vi "Gage_Set.vi"(7 "Scope":bool, 10 "Handle Cluster 2":T1, 11 "Handle Cluster 1":T1) -> (0 "Waveform Graph":cluster{i32, dbl, dbl[]}(graph), 1 "Equivalent RT delay\ndistance (mm)":dbl=1.5 format="%.4f")   [LabVIEW 2022 SP3]
uses:
  <vilib>/Analysis/NI_AALPro.lvlib
  -GageUtils/GageGlobals.vi
  <vilib>/Utility/file.llb/Write To Spreadsheet File (DBL).vi
  <vilib>/Analysis/NI_AALBase.lvlib
  <vilib>/Analysis/baseanly.llb/Mean (DBL).vi
panel:
  in  "Slave scales":bool
  in  "holdoff (ms)":dbl min=0.0
  out "Gage Chan 9-16":dbl[][](graph)
  out "LeCroy Ch1":dbl[](graph)
  in  "Set LeCroy":bool
  in  "time out (ms)":dbl=1000.0 min=-1.0
  in  "Vpp Chs 2":i16[](array[ring])=[5, 5, 5, 5, 5, 5, 5, 5]
  in  "Ch":u16 max=15
  out "Status":string
  in  "Mode":u16(ring)=3 items=["Single", "Dual", "Quad", "Octal"]
  in  "Coupling":u16(ring) items=["DC", "AC"]
  in  "Impedance":u32=50 min=50 max=1000000 step=999950
  out "Nominal Samples":i32
  out "t per div":dbl
  in  "Vpp Chs 1":i16[](array[ring])=[5, 5, 5, 5, 5, 5, 5, 5]
  out "Gage Chan 1-8":dbl[][](graph)
  in  "Save trace?":bool
  out "Total Delay (ms)":dbl=1.5 format="%.3f"
  in  "go to scan type":bool
  in  "ExitSendCmd":bool
  in  "Time scale per Div":i32(ring)=1 items=["1 micros", "2 micros", "5 micros", "10 micros", "20 micros", "50 micros", "100 micros", "200 micros", "500 micros", "1 ms", "2 ms", "5 ms", "10 ms"]
  in  "Trigger Settings":T2={"Trig Source"=1, "Level (%)"=25.0, "External"=TRUE, "Ext Impedance"=1, "External Coupling"=0, "Ext Trig Range"=0, "Slope"=0} {"Slope" items=["Rising", "Falling"]; "Ext Trig Range" items=["+/- 5 Volts", "+/- 1 Volt"]; "External Coupling" items=["DC", "AC"]; "Ext Impedance" items=["50 Ohm", "HiZ"]; "Level (%)" min=-100.0 max=100.0 format="%#.2f"; "Trig Source" items=["Ch 0", "Ch 1", "Ch 2", "Ch 3", "Ch 4", "Ch 5", "Ch 6", "Ch 7"]}
  in  "RF data Sampling":T3={"Sampling Rate"=6, "Ref Delay (ms)"=0.0, "rf points per line"=2048} {"Sampling Rate" items=["1 MS/s", "5 MS/s", "10 MS/s", "25 MS/s", "50 MS/s", "100 MS/s", "125 MS/s"]; "Ref Delay (ms)" min=0.0 format="%.2f"}
  # "Digitizer Settings"
  # "Scale Settings"
  # "Yellow curser used for additional delay. RF data is captured between yellow and red lines."
  # "Scope sampling rate should be fixed at 250 MS/s"
  # "© 2009 Riverside Research Institute"
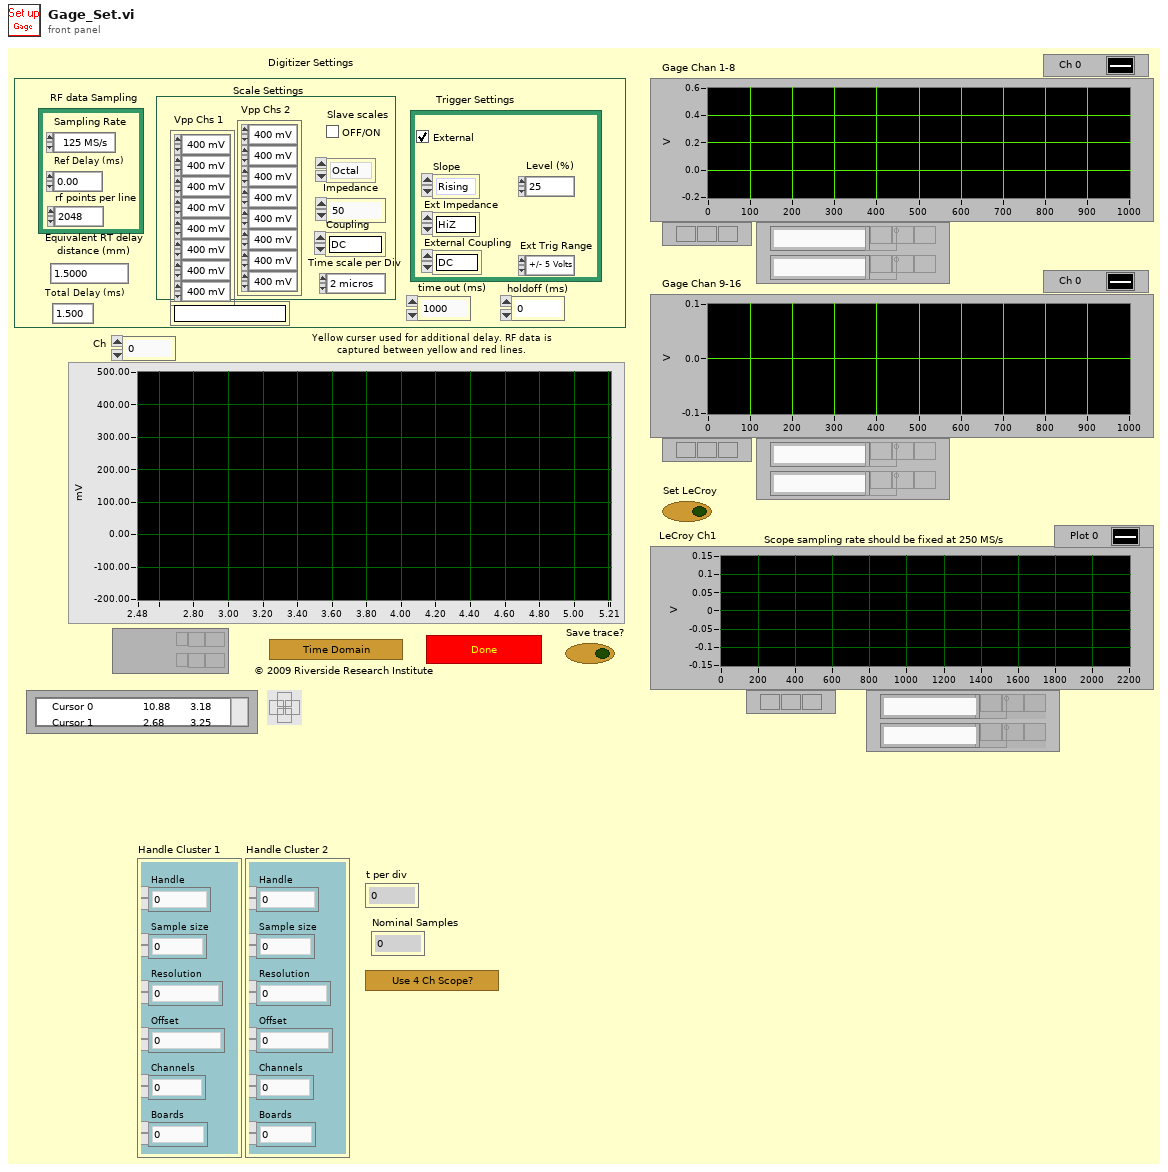
[diagram p1: front panel]
types:
  T1 = cluster{"Handle":u32, "Sample size":u32, "Resolution":i32, "Offset":i32, "Channels":u32, "Boards":u32}
  T2 = cluster{"Trig Source":u16, "Level (%)":dbl, "External":bool, "Ext Impedance":u16, "External Coupling":u16, "Ext Trig Range":i16, "Slope":u16}
  T3 = cluster{"Sampling Rate":u16, "Ref Delay (ms)":dbl, "rf points per line":i32}
  T4 = cluster{"Handle":u32, "Sample Size":u32, "Resolution":i32, "Offset":i32, "Channels":u32, "Boards":u32}
  T5 = cluster{dbl, "Clock mode":enum16{"Internal", "External", "Reference"}, "RingText.Text":string, i32, i32, "time out (ms)":dbl, dbl, dbl}
  T6 = cluster{"RingText.Text":string, bool, bool, i16, "Impedance":u32, i32, i32}
  T7 = cluster{"RingText.Text":string, "Level (%)":dbl, "Trig Source":u16, i32, "RingText.Text":string, "External":bool, bool, "RingText.Text":string}
  T8 = cluster{"RingText.Text":string, "Level (%)":dbl, "Trig Source":u16, i32, "RingText.Text":string, "External":bool, bool, "RingText.Text":string}[]
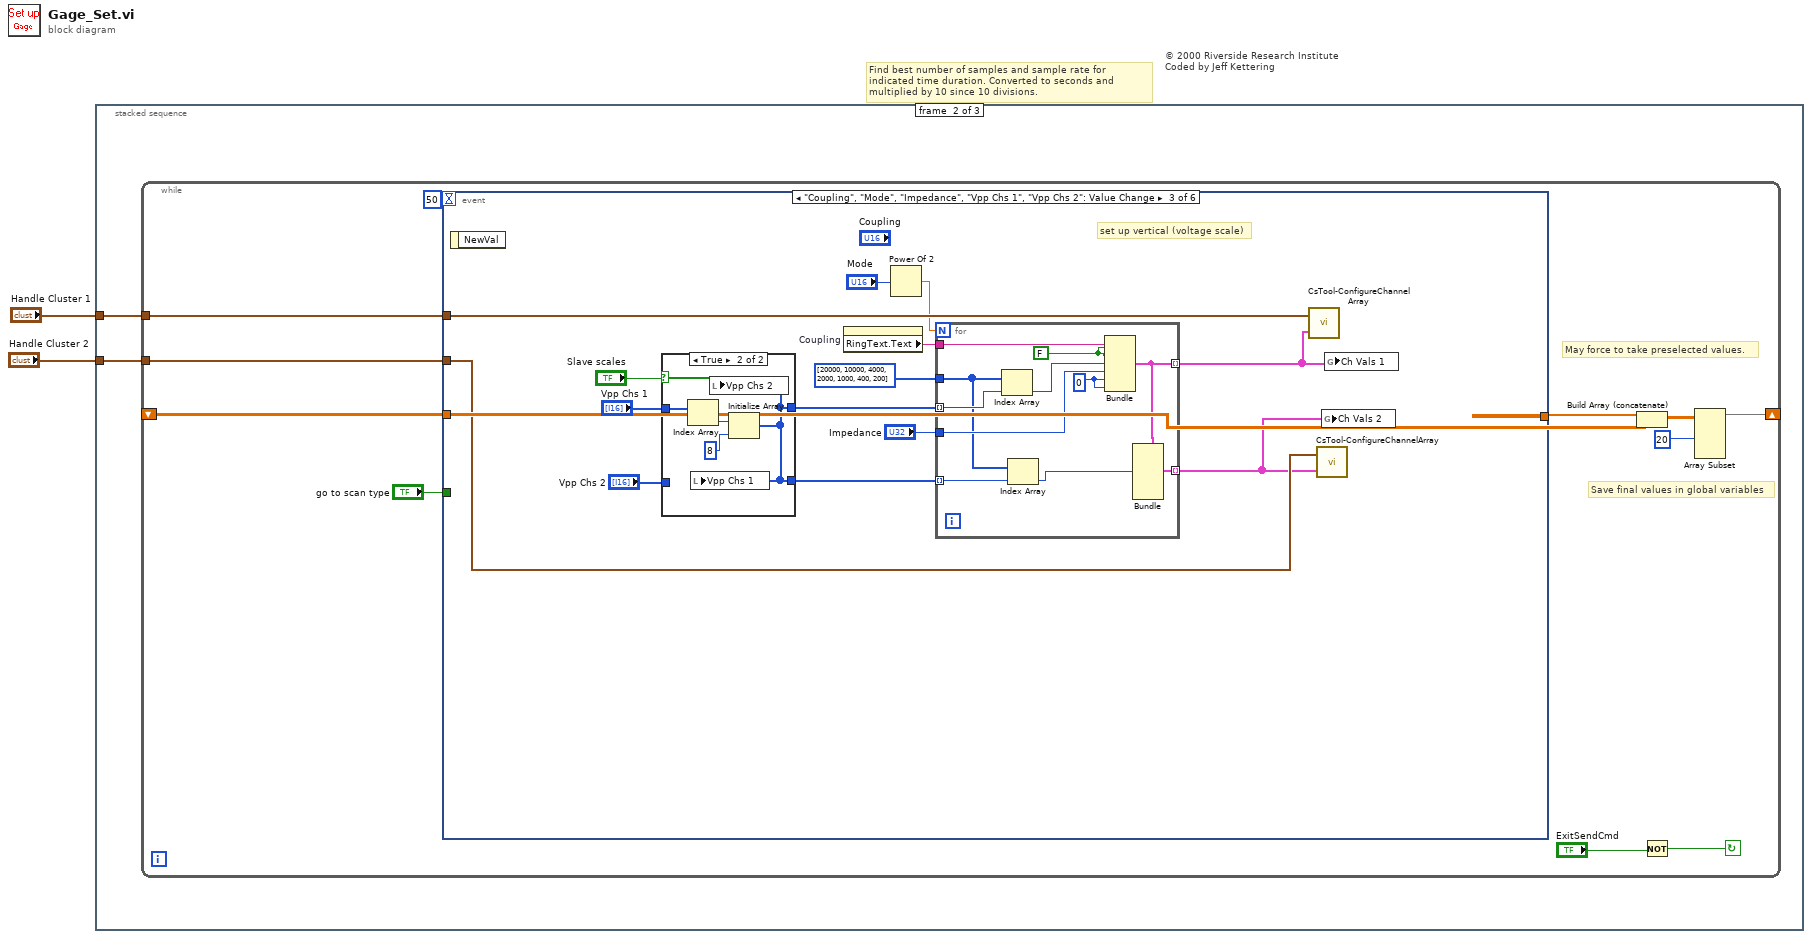
[diagram p0: block diagram]
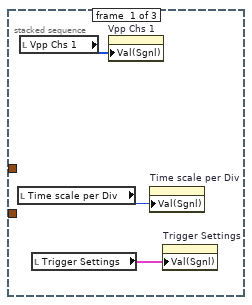
[diagram p2: hidden frame]
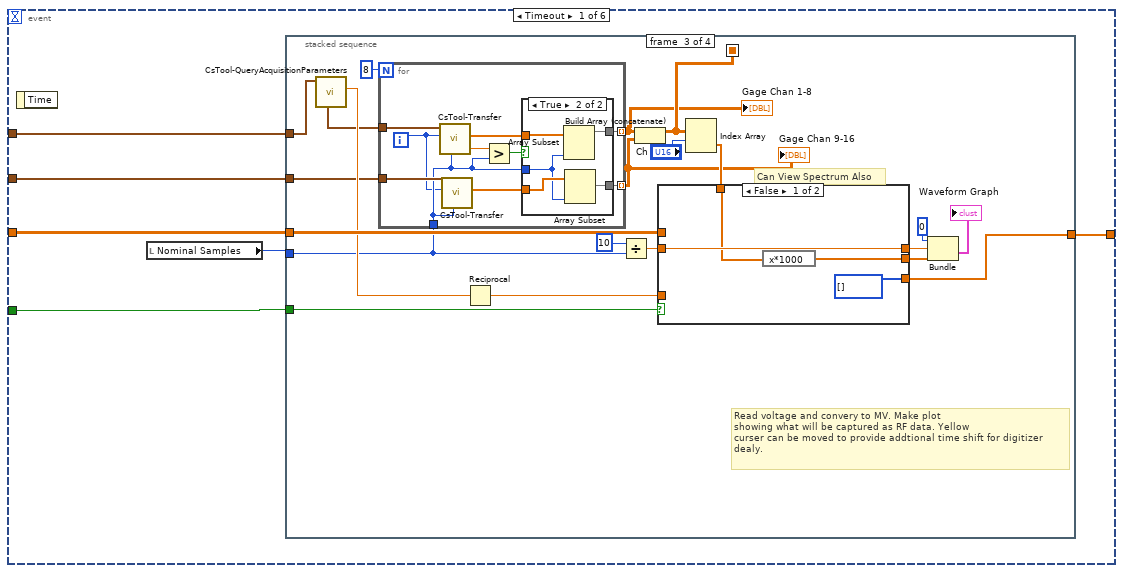
[diagram p3: hidden frame]
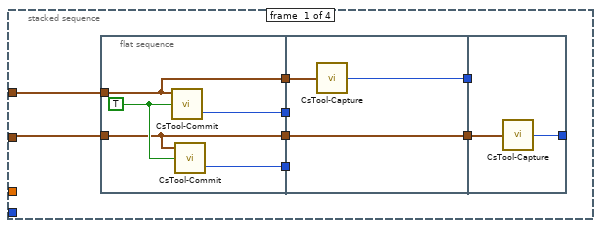
[diagram p4: hidden frame]
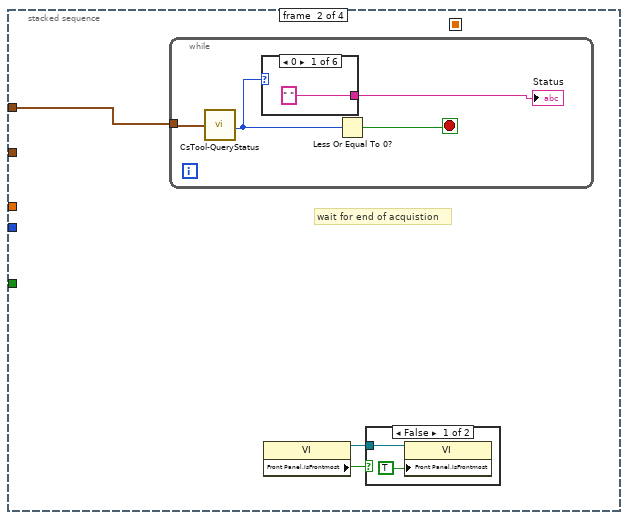
[diagram p5: hidden frame]
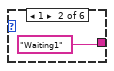
[diagram p6: hidden frame]
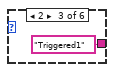
[diagram p7: hidden frame]
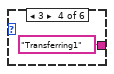
[diagram p8: hidden frame]
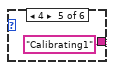
[diagram p9: hidden frame]
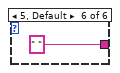
[diagram p10: hidden frame]
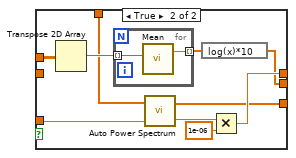
[diagram p13: hidden frame]
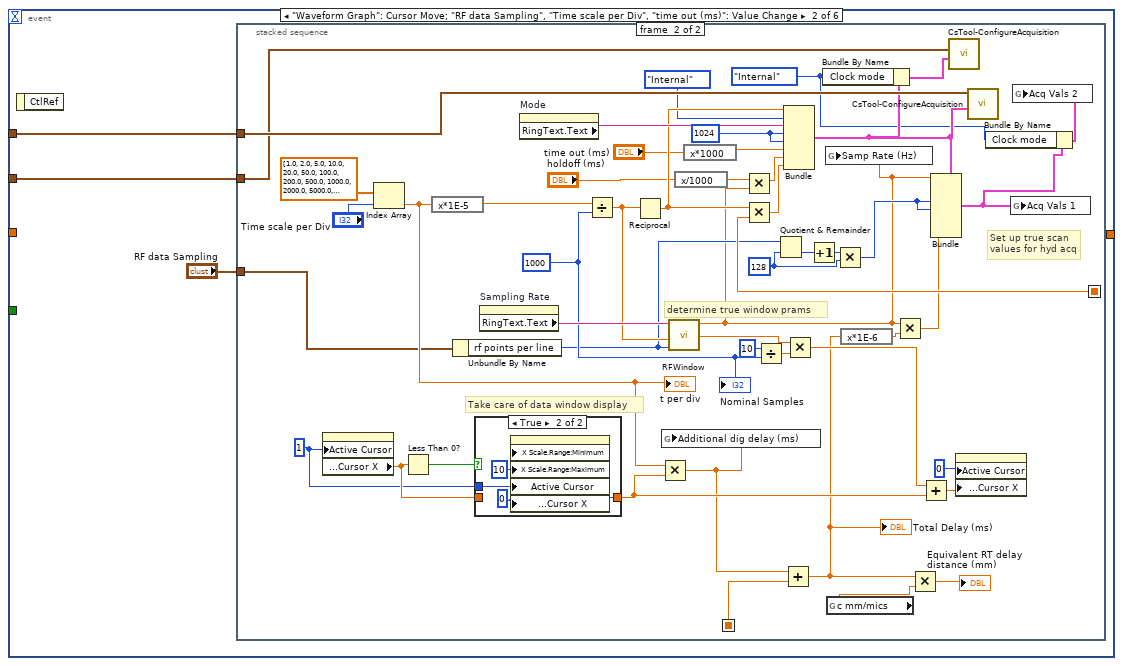
[diagram p15: hidden frame]
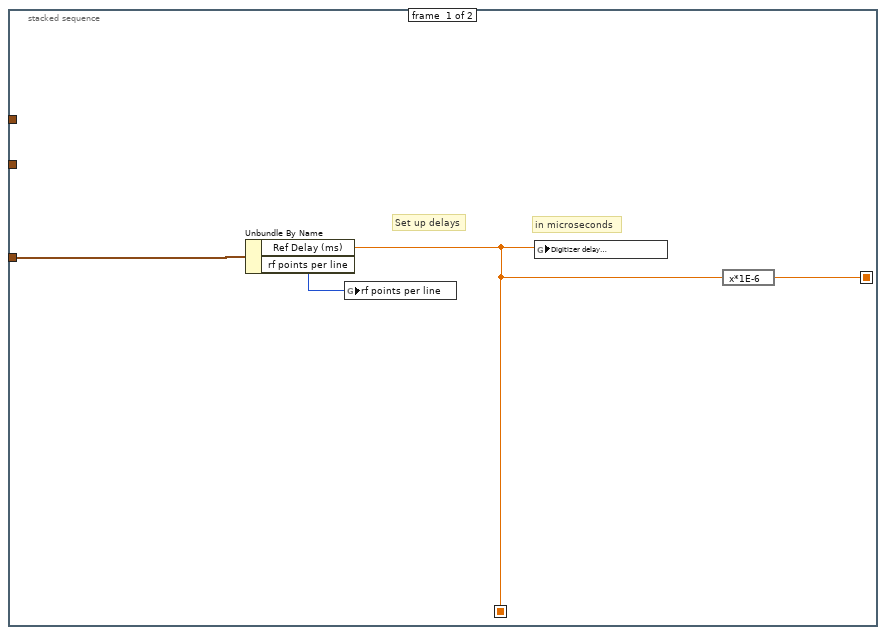
[diagram p16: hidden frame]
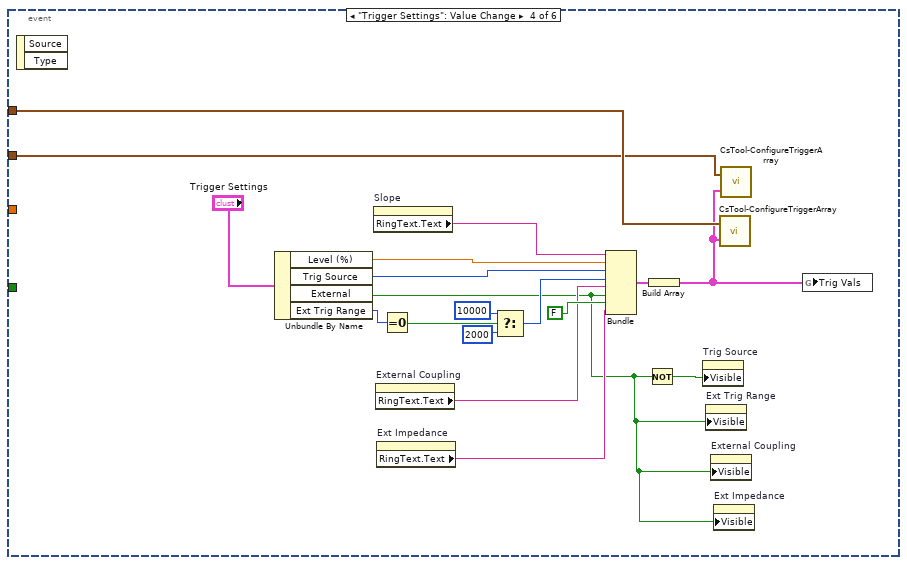
[diagram p19: hidden frame]
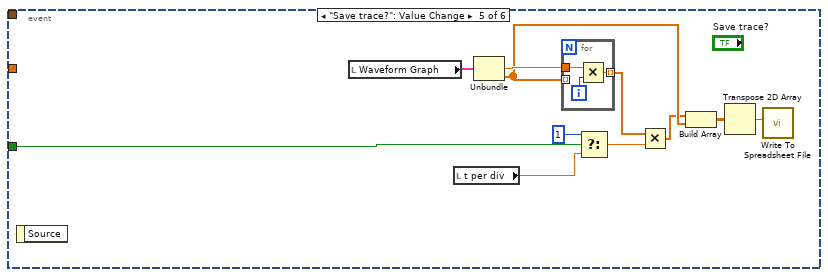
[diagram p20: hidden frame]
diagram:
  # "Find best number of samples and sample rate for indicated time duration. Converted to seconds and multiplied by 10 since 10 divisions."
  # "© 2000 Riverside Research Institute\nCoded by Jeff Kettering"
  n1 = stacked-sequence {
    tunnel: "Handle Cluster 1" -> [_ w7 _]
    tunnel: "Handle Cluster 2" -> [_ w6 _]
    frame #0 {
      n2 = local read "Time scale per Div"() -> (w4:i32)
      n3 = local read "Vpp Chs 1"() -> (w5:i16[])
      n4 = local read "Trigger Settings"() -> (w3:T2)
      n5 = property on="Vpp Chs 1" class="Arr (strict)"("Val(Sgnl)"=w5) -> ()  [unwired: 2 in, 2 out]
      n6 = property on="Time scale per Div" class="Ring (strict)"("Val(Sgnl)"=w4) -> ()  [unwired: 2 in, 2 out]
      n7 = property on="Trigger Settings" class="Clust (strict)"("Val(Sgnl)"=w3) -> ()  [unwired: 2 in, 2 out]
    }
    frame #1 {
      n8 = while {
        shift-left: _ -> [w9]
        shift-right: [w14] -> _
        tunnel: w7 -> [w11]
        tunnel: w6 -> [w8]
        stop <- w17 continue-if-true
        # "May force to take preselected values."
        # "Save final values in global variables"
        n9 = event shown="[2] \"Coupling\", \"Mode\", \"Impedance\", \"Vpp Chs 1\", \"Vpp Chs 2\": Value Change" {
          selector: _ -> [_ _ _ _ _ _]
          dyn-events: _ -> [_ _ _ _ _ _]
          timeout: 50 -> [_ _ _ _ _ _]
          tunnel: "go to scan type" -> [w22 _ _ _ w223 _]
          tunnel: w11 -> [w21 w114 w185 w219 _ _]
          tunnel: w9 -> [w24 _ _ _ _ _]
          tunnel: [w23 _ _ _ _ _] -> w16
          tunnel: w8 -> [w19 w112 w178 w205 _ _]
          event Timeout {
            n10 = event-data() -> ()  [unwired: 2 out]
            n11 = local read "Nominal Samples"() -> (w20:i32)
            n12 = stacked-sequence {
              seq-local: [_ _ w61 _] -> [_ _ _ _]
              tunnel: w21 -> [w32 w43 w64 _]
              tunnel: w24 -> [_ _ w73 _]
              tunnel: [_ _ w72 _] -> w23
              tunnel: w22 -> [_ _ w71 _]
              tunnel: w20 -> [_ _ w65 _]
              tunnel: w19 -> [w26 _ w60 _]
              frame #0 {
                n13 = flat-sequence {
                  tunnel: w32 -> [w35]
                  tunnel: [w35] -> w31
                  tunnel: [w37] -> w30
                  tunnel: [w36] -> w29
                  tunnel: [w33] -> w27
                  tunnel: w26 -> [w33]
                  tunnel: w31 -> [w40]
                  tunnel: w30 -> [_]
                  tunnel: w29 -> [_]
                  tunnel: [w39] -> w28
                  tunnel: w27 -> [w39]
                  tunnel: [w38] -> w25
                  tunnel: w28 -> [w42]
                  tunnel: w25 -> [_]
                  tunnel: [w41] -> _
                  frame #0 {
                    w34 = TRUE ("Coerce Flag (f)")
                    n14 = call <userlib>:"CsTool-Commit.vi"("Coerce Flag (f)"=w34, "Handle Cluster"=w35) -> ("Error Code"=w37:i32)  [unwired: 1 in, 1 out]
                    n15 = call <userlib>:"CsTool-Commit.vi"("Coerce Flag (f)"=w34, "Handle Cluster"=w33) -> ("Error Code"=w36:i32)  [unwired: 1 in, 1 out]
                  }
                  frame #1 {
                    n16 = call <userlib>:"CsTool-Capture.vi"("Handle Cluster"=w40) -> ("Error Code"=w38:i32)
                  }
                  frame #2 {
                    n17 = call <userlib>:"CsTool-Capture.vi"("Handle Cluster"=w42) -> ("Error Code"=w41:i32)
                  }
                }
              }
              frame #1 {
                # "wait for end of acquistion"
                n18 = while {
                  tunnel: w43 -> [w48]
                  stop <- w47 stop-if-true
                  n19 = call <userlib>:"CsTool-QueryStatus.vi"("Handle Cluster"=w48) -> ("Status"=w49:i32)
                  n20 = case shown="0" w49 {
                    tunnel: [" " "Waiting1" "Triggered1" "Transferring1" "Calibrating1" " "] -> w46
                    frame 0 {
                    }
                    frame 1 {
                    }
                    frame 2 {
                    }
                    frame 3 {
                    }
                    frame 4 {
                    }
                    frame 5, Default {
                    }
                  }
                  "Status" <- w46
                  n21 = Less Or Equal To 0?(x=w49) -> (x <= 0?=w47:bool)
                }
                n22 = property class="VI"() -> (reference out=w45:refnum<vi>, "Front Panel.IsFrontmost"=w44:bool)  [unwired: 2 in, 1 out]
                n23 = case shown="False" w44 {
                  tunnel: w45 -> [w57 _]
                  frame False {
                    n24 = property class="VI"(reference=w57, "Front Panel.IsFrontmost"=TRUE) -> ()  [unwired: 1 in, 2 out]
                  }
                  frame True {
                  }
                }
              }
              frame #2 {
                # "Can View Spectrum Also"
                # "Read voltage and convery to MV. Make plot\nshowing what will be captured as RF data. Yellow\ncurser can be moved to provide addtional time shift for digitizer\ndealy."
                n25 = call <userlib>:"CsTool-QueryAcquisitionParameters.vi"("Handle Cluster"=w64) -> ("Output Handle Cluster"=w63:T4, "Sample Rate"=w67:dbl)  [unwired: 9 out]
                n26 = for {
                  N: 8 -> [_]
                  tunnel: [w87] -> w59 mode=indexing
                  tunnel: w63 -> [w86]
                  tunnel: w65 -> [w83]
                  tunnel: w60 -> [w84]
                  tunnel: [w82] -> w58 mode=indexing
                  i -> [w81]
                  n27 = call <userlib>:"CsTool-Transfer.vi"("Length (4096)"=w83, "Channel (0)"=w81, "Handle Cluster"=w86) -> ("Actual Length"=w85:dbl, "Data in Volts"=w79:dbl[])  [unwired: 3 in, 2 out]
                  n28 = call <userlib>:"CsTool-Transfer.vi"("Length (4096)"=w83, "Channel (0)"=w81, "Handle Cluster"=w84) -> ("Data in Volts"=w80:dbl[])  [unwired: 3 in, 3 out]
                  n29 = Greater?(x=w85, y=w83) -> (0:w88:bool)
                  n30 = case shown="True" w88 {
                    tunnel: w79 -> [w90 w95]
                    tunnel: [w90 w94] -> w87
                    tunnel: w83 -> [_ w91]
                    tunnel: w80 -> [w89 w93]
                    tunnel: [w89 w92] -> w82
                    frame False {
                    }
                    frame True {
                      n31 = Array Subset(array=w95, length=w91) -> (w94:dbl[])  [unwired: 1 in]
                      n32 = Array Subset(array=w93, length=w91) -> (w92:dbl[])  [unwired: 1 in]
                    }
                  }
                }
                "Gage Chan 1-8" <- w59
                "Gage Chan 9-16" <- w58
                n33 = Reciprocal(x=w67) -> (1/x=w66:dbl)
                n34 = Divide(x=10, y=w65) -> (x/y=w75:dbl)
                n35 = Build Array (concatenate)(w59, w58) -> (w61:dbl[][])
                n36 = Index Array(array=w61, index (row)="Ch") -> (element=w68:dbl[])  [unwired: 1 in]
                n37 = case shown="False" w71 {
                  tunnel: [w96 w101] -> w70
                  tunnel: w68 -> [w97 w107]
                  tunnel: [w99 w103] -> w76
                  tunnel: w75 -> [w99 _]
                  tunnel: w73 -> [_ w106]
                  tunnel: w66 -> [_ w105]
                  tunnel: [i32[] [] w102] -> w72
                  frame False {
                    n38 = expression code="x*1000"(w97) -> (w96:dbl[])
                  }
                  frame True {
                    n39 = Transpose 2D Array(2D array=w106) -> (transposed array=w108:dbl[][])
                    n40 = for {
                      tunnel: w108 -> [w111] mode=indexing
                      tunnel: [w110] -> w100 mode=indexing
                      n41 = call-poly <vilib>:"Mean.vi"("X"=w111) -> ("mean"=w110:dbl)  [unwired: 1 out]
                    }
                    n42 = call <vilib>:"Auto Power Spectrum.vi"("dt"=w105, "Signal (V)"=w107) -> ("df"=w104:dbl, "Power Spectrum (V^2 rms)"=w102:dbl[])
                    n43 = expression code="log(x)*10"(w100) -> (w101:dbl[])
                    n44 = Multiply(x=w104, y=1e-06) -> (x*y=w103:dbl)
                  }
                }
                n45 = Bundle(0, w76, w70) -> (→"Waveform Graph":cluster{i32, dbl, dbl[]})  [unwired: 1 out]
              }
              frame #3 {
                # "May need to alter display to break into subplots"
              }
            }
          }
          event "Waveform Graph": Cursor Move; "RF data Sampling", "Time scale per Div", "time out (ms)": Value Change {
            n46 = event-data() -> ()  [unwired: 2 out]
            n47 = stacked-sequence {
              seq-local: [w118 _] -> [_ w145]
              seq-local: [w116 _] -> [_ w157]
              tunnel: w114 -> [_ w148]
              tunnel: "RF data Sampling" -> [w117 w152]
              tunnel: w112 -> [_ w133]
              frame #0 {
                # "Set up delays"
                # "in microseconds"
                n48 = Unbundle By Name(w117) -> ("Ref Delay (ms)"=w116:dbl, "rf points per line"=w115:i32)
                n49 = global write "GageGlobals.vi" "rf points per line"(w115) -> ()
                n50 = global write "GageGlobals.vi" "Digitizer delay\n (ms)"(w116) -> ()
                n51 = expression code="x*1E-6"(w116) -> (w118:dbl)
              }
              frame #1 {
                w124 = enum16{"Internal", "External", "Reference"}."Internal" ("Clock mode")
                w137 = 128
                w144 = 1024
                w143 = 1000
                w163 = u32 1 ("Write Attribute")
                # "determine true window prams"
                # "Set up true scan values for hyd acq"
                # "Take care of data window display"
                n52 = property on="Waveform Graph" class="WFGraph (strict)"("Active Cursor"=w163) -> ("Cursor.Cursor Position:Cursor X"=w165:dbl)  [unwired: 2 in, 2 out]
                n53 = Index Array(array=dbl[] [1.0, 2.0, 5.0, 10.0, 20.0, 50.0, 100.0, 200.0, 500.0, 1000.0, 2000.0, 5000.0, 10000.0, 20000.0, 50000.0, 100000.0], index="Time scale per Div") -> (element=w154:dbl)
                "t per div" <- w154
                n54 = Less Than 0?(x=w165) -> (x < 0?=w164:bool)
                n55 = expression code="x*1E-5"(w154) -> (w150:dbl)
                n56 = Unbundle By Name(w152) -> ("rf points per line"=w135:i32)
                n57 = case shown="True" w164 {
                  tunnel: w165 -> [w168 _]
                  tunnel: [w168 w169] -> w160
                  tunnel: w163 -> [_ w171]
                  frame False {
                  }
                  frame True {
                    w169 = 0
                    n58 = property on="Waveform Graph" class="WFGraph (strict)"("X Scale.Range:Minimum"=w169, "X Scale.Range:Maximum"=10, "Active Cursor"=w171, "Cursor.Cursor Position:Cursor X"=w169) -> ()  [unwired: 2 in, 2 out]
                  }
                }
                n59 = property on="Sampling Rate" class="Ring (strict)"() -> ("RingText.Text"=w151:string)  [unwired: 2 in, 2 out]
                n60 = property on="Mode" class="Ring (strict)"() -> ("RingText.Text"=w147:string)  [unwired: 2 in, 2 out]
                n61 = Divide(x=w150, y=w143) -> (x/y=w149:dbl)
                n62 = Reciprocal(x=w149) -> (1/x=w142:dbl)
                n63 = Multiply(x=w154, y=w160) -> (x*y=w130:dbl)
                n64 = global write "GageGlobals.vi" "Additional dig delay (ms)"(w130) -> ()
                n65 = call "RFWindow.vi"("rf points per line"=w135, "Sample Time"=w149, "Text of Samp Rate"=w151) -> ("curser position"=w158:dbl, "Sampling (Hz)"=w119:dbl)  [unwired: 1 in, 2 out]
                n66 = expression code="x/1000"("holdoff (ms)") -> (w121:dbl)
                n67 = expression code="x*1000"("time out (ms)") -> (w131:dbl)
                n68 = Multiply(x=w121, y=w119) -> (x*y=w120:dbl)
                n69 = Multiply(x=w142, y=w145) -> (x*y=w146:dbl)
                n70 = Divide(x=10, y=w143) -> (x/y=w159:dbl)
                n71 = Quotient & Remainder(x=w135, y=w137) -> (floor(x/y)=w136:i32)  [unwired: 1 out]
                n72 = Add(x=w130, y=w157) -> (x+y=w139:dbl)
                "Total Delay (ms)" <- w139
                n73 = Bundle(w142, "Clock mode"=enum16{"Internal", "External", "Reference"}."Internal", "RingText.Text"=w147, w144, w144, "time out (ms)"=w131, w120, w146) -> (w128:T5)  [unwired: 1 out]
                n74 = Multiply(x=w158, y=w159) -> (x*y=w161:dbl)
                n75 = Increment(x=w136) -> (x+1=w138:i32)
                n76 = Bundle By Name(cluster=w128, "Clock mode"=w124) -> (w126:T5)
                n77 = global write "GageGlobals.vi" "Samp Rate (Hz)"(w119) -> ()
                n78 = global read "GageGlobals.vi" "c mm/mics"() -> (w129:sgl)
                n79 = Multiply(x=w138, y=w137) -> (x*y=w134:i32)
                n80 = expression code="x*1E-6"(w139) -> (w140:dbl)
                n81 = Multiply(x=w119, y=w140) -> (x*y=w141:dbl)
                n82 = Multiply(x=w139, y=w129) -> (x*y=→"Equivalent RT delay\ndistance (mm)":dbl)
                n83 = Add(x=w161, y=w160) -> (x+y=w162:dbl)
                n84 = Bundle(cluster=w128, w119, w134, w134, w141) -> (w125:T5)  [unwired: 4 out]
                n85 = call <userlib>:"CsTool-ConfigureAcquisition.vi"("Handle Cluster"=w133, "Acquisition"=w126) -> ()  [unwired: 3 in, 1 out]
                n86 = property on="Waveform Graph" class="WFGraph (strict)"("Active Cursor"=u32 0, "Cursor.Cursor Position:Cursor X"=w162) -> ()  [unwired: 2 in, 2 out]
                n87 = call <userlib>:"CsTool-ConfigureAcquisition.vi"("Handle Cluster"=w148, "Acquisition"=w128) -> ()  [unwired: 3 in, 1 out]
                n88 = Bundle By Name(cluster=w125, "Clock mode"=w124) -> (w123:T5)
                n89 = global write "GageGlobals.vi" "Acq Vals 1"(w125) -> ()
                n90 = global write "GageGlobals.vi" "Acq Vals 2"(w123) -> ()
                "Nominal Samples" <- w143
              }
            }
          }
          event "Coupling", "Mode", "Impedance", "Vpp Chs 1", "Vpp Chs 2": Value Change {
            # "set up vertical (voltage scale)"
            n91 = event-data() -> ()  [unwired: 2 out]
            n92 = case shown="True" "Slave scales" {
              tunnel: "Vpp Chs 1" -> [w187 w189]
              tunnel: [w187 w188] -> w174
              tunnel: [w186 w188] -> w172
              tunnel: "Vpp Chs 2" -> [w186 _]
              frame False {
              }
              frame True {
                n93 = Index Array(array=w189) -> (element=w190:i16)  [unwired: 1 in]
                n94 = Initialize Array(w190, 8) -> (w188:i16[])
                n95 = local write "Vpp Chs 1"(w188) -> ()
                n96 = local write "Vpp Chs 2"(w188) -> ()
              }
            }
            n97 = property on="Coupling" class="Ring (strict)"() -> ("RingText.Text"=w184:string)  [unwired: 2 in, 2 out]
            n98 = Power Of 2(x="Mode") -> (2^x=w180:dbl)
            n99 = for {
              N: w180 -> [_]
              tunnel: w184 -> [w202]
              tunnel: i16[] [20000, 10000, 4000, 2000, 1000, 400, 200] -> [w196]
              tunnel: "Impedance" -> [w199]
              tunnel: w174 -> [w197] mode=indexing
              tunnel: [w193] -> w179 mode=indexing
              tunnel: w172 -> [w195] mode=indexing
              tunnel: [w192] -> w177 mode=indexing
              w198 = 0
              w201 = FALSE
              n100 = Index Array(array=w196, index=w197) -> (element=w200:i16)
              n101 = Index Array(array=w196, index=w195) -> (element=w194:i16)
              n102 = Bundle("RingText.Text"=w202, w201, w201, w200, "Impedance"=w199, w198, w198) -> (w193:T6)  [unwired: 1 out]
              n103 = Bundle(cluster=w193, w194) -> (w192:T6)  [unwired: 6 out]
            }
            n104 = call <userlib>:"CsTool-ConfigureChannelArray.vi"("Channels"=w179, "Handle Cluster"=w185) -> ()  [unwired: 1 out]
            n105 = call <userlib>:"CsTool-ConfigureChannelArray.vi"("Channels"=w177, "Handle Cluster"=w178) -> ()  [unwired: 1 out]
            n106 = global write "GageGlobals.vi" "Ch Vals 2"(w177) -> ()
            n107 = global write "GageGlobals.vi" "Ch Vals 1"(w179) -> ()
          }
          event "Trigger Settings": Value Change {
            n108 = event-data() -> ()  [unwired: 3 out]
            n109 = Unbundle By Name("Trigger Settings") -> ("Level (%)"=w215:dbl, "Trig Source"=w214:u16, "External"=w203:bool, "Ext Trig Range"=w211:i16)
            n110 = property on="Slope" class="Ring (strict)"() -> ("RingText.Text"=w212:string)  [unwired: 2 in, 2 out]
            n111 = property on="External Coupling" class="Ring (strict)"() -> ("RingText.Text"=w213:string)  [unwired: 2 in, 2 out]
            n112 = property on="Ext Impedance" class="Ring (strict)"() -> ("RingText.Text"=w216:string)  [unwired: 2 in, 2 out]
            n113 = Equal To 0?(x=w211) -> (x = 0?=w210:bool)
            n114 = Select(t=10000, s=w210, f=2000) -> (s? t:f=w207:i32)
            n115 = Bundle("RingText.Text"=w212, "Level (%)"=w215, "Trig Source"=w214, w207, "RingText.Text"=w213, "External"=w203, FALSE, "RingText.Text"=w216) -> (w218:T7)  [unwired: 1 out]
            n116 = Not(x=w203) -> (.not. x?=w204:bool)
            n117 = Build Array(w218) -> (w206:T8)
            n118 = property on="Trig Source" class="Ring (strict)"("Visible"=w204) -> ()  [unwired: 2 in, 2 out]
            n119 = property on="Ext Trig Range" class="Ring (strict)"("Visible"=w203) -> ()  [unwired: 2 in, 2 out]
            n120 = property on="External Coupling" class="Ring (strict)"("Visible"=w203) -> ()  [unwired: 2 in, 2 out]
            n121 = property on="Ext Impedance" class="Ring (strict)"("Visible"=w203) -> ()  [unwired: 2 in, 2 out]
            n122 = call <userlib>:"CsTool-ConfigureTriggerArray.vi"("Triggers"=w206, "Handle Cluster"=w219) -> ()  [unwired: 1 out]
            n123 = call <userlib>:"CsTool-ConfigureTriggerArray.vi"("Triggers"=w206, "Handle Cluster"=w205) -> ()  [unwired: 1 out]
            n124 = global write "GageGlobals.vi" "Trig Vals"(w206) -> ()
          }
          event "Save trace?": Value Change {
            n125 = event-data() -> ()  [unwired: 2 out]
            n126 = local read "Waveform Graph"() -> (w222:cluster{i32, dbl, dbl[]})
            n127 = local read "t per div"() -> (w221:dbl)
            n128 = Unbundle(w222) -> (w231:dbl, w230:dbl[])  [unwired: 1 out]
            n129 = for {
              tunnel: w231 -> [w233]
              tunnel: w230 -> [_] mode=indexing
              tunnel: [w232] -> w227 mode=indexing
              i -> [w234]
              n130 = Multiply(x=w233, y=w234) -> (x*y=w232:dbl)
            }
            n131 = Select(t=1, s=w223, f=w221) -> (s? t:f=w224:dbl)
            n132 = Multiply(x=w227, y=w224) -> (x*y=w226:dbl[])
            n133 = Build Array(w226, w230) -> (w229:dbl[][])
            n134 = Transpose 2D Array(2D array=w229) -> (transposed array=w228:dbl[][])
            n135 = call-poly <vilib>:"Write To Spreadsheet File.vi"("2D data"=w228) -> ()  [unwired: 5 in, 3 out]
          }
          event "Set LeCroy": Value Change {
            n136 = event-data() -> ()  [unwired: 7 out]
            n137 = call "LecroySet.vi"() -> ("Test Waveorm"=→"LeCroy Ch1":dbl[])  [unwired: 1 in, 10 out]
          }
        }
        n138 = Build Array (concatenate)(w16, w9) -> (w15:dbl[][])
        n139 = Not(x="ExitSendCmd") -> (.not. x?=w17:bool)
        n140 = Array Subset(array=w15, length (row)=20) -> (w14:dbl[][])  [unwired: 3 in]
      }
    }
    frame #2 {
      n141 = case shown="True" "Scope" {
        frame False {
        }
        frame True {
          n142 = call "LecroySet.vi"() -> ()  [unwired: 1 in, 11 out]
        }
      }
    }
  }
